vi "Start logging.vi"(3 "Custom rate":dbl=8.0, 4 "File Segmenting size (MB)":dbl=8.0, 5 "custom logging rate?":bool, 6 "FilePropertyValues":string[](array[string]), 7 "Segment Files? (F)":bool, 8 "FilePropertyNames":string[](array[string]), 9 "File Description":string, 10 "Channel paths":string[](array[string])=["Aliases/ActualRPM", "Aliases/DesiredRPM", "Aliases/EnginePower", "Aliases/EngineTemp"], 11 "Base Log File Path":path=path "C:/Users/aheim/Desktop/test.tdms") -> (0 "error out":errorcluster, 1 "Report Text":string)   [LabVIEW 2013, in "Logger.lvlib"]
uses:
  Logger.lvlib
  <vilib>/NI Veristand/Execution/DataLogging/File Conflict Operation.ctl
  <vilib>/NI Veristand/Execution/DataLogging/TDMS Channel Group.ctl
  <vilib>/NI Veristand/Execution/DataLogging/TDMS Property.ctl
  <vilib>/NI Veristand/Execution/DataLogging/TDMS Channel.ctl
  <vilib>/NI Veristand/Execution/DataLogging/Time Channel Options.ctl
  <vilib>/NI Veristand/Execution/DataLogging/New Data Logging Specification (TDMS).vi
  <vilib>/NI Veristand/Execution/DataLogging/Set Data Logging Rate (Target Rate).vi
  <vilib>/NI Veristand/Execution/DataLogging/Set Data Logging Rate (Custom Rate).vi
  <vilib>/NI Veristand/Execution/DataLogging/Set Segmenting Specification (Footprint).vi
  <vilib>/NI Veristand/Execution/DataLogging/NI_VS Data Logging API.lvlib
panel:
  in  "Gateway IP Address (\"\": localhost)":string
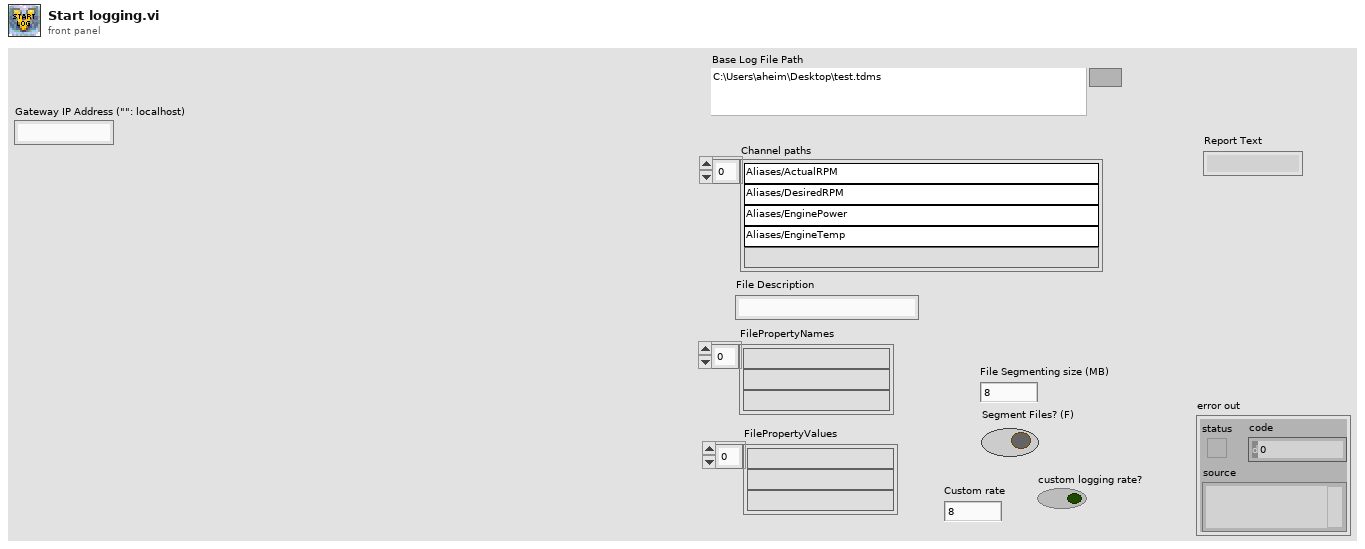
[diagram p1: front panel]
types:
  T1 = typedef "NI_VS Data Logging API.lvlib/Time Channel Options.ctl" = enum16{"No Time Channel", "Absolute Time", "System Time", "System Time - Microseconds", "Absolute Time as Double"}
  T2 = typedef "NI_VS Data Logging API.lvlib/TDMS Channel Group.ctl" = cluster{"Group Name":string, "Group Description":string, "Group Properties":T3[], "Channels":T4[], "Time Channel Options":T1, "Time Channel Name":string}
  T3 = typedef "NI_VS Data Logging API.lvlib/TDMS Property.ctl" = cluster{"Name":string, "Value":variant}
  T4 = typedef "NI_VS Data Logging API.lvlib/TDMS Channel.ctl" = cluster{"Channel Name":string, "Channel Path":string, "Channel Description":string, "Channel Properties":T3[]}
  T5 = typedef "NI_VS Data Logging API.lvlib/File Conflict Operation.ctl" = enum16{"Create Unique", "Append to Existing", "Overwrite"}
  T6 = cluster{"PropertyName":string, "PropertyValue":string}
  T7 = typedef "NI_VS Data Logging API.lvlib/IDataLogging Ref.ctl" = refnum<k24>
  T8 = typedef "NI_VS Data Logging API.lvlib/DataLoggingSpecification Ref.ctl" = refnum<k24>
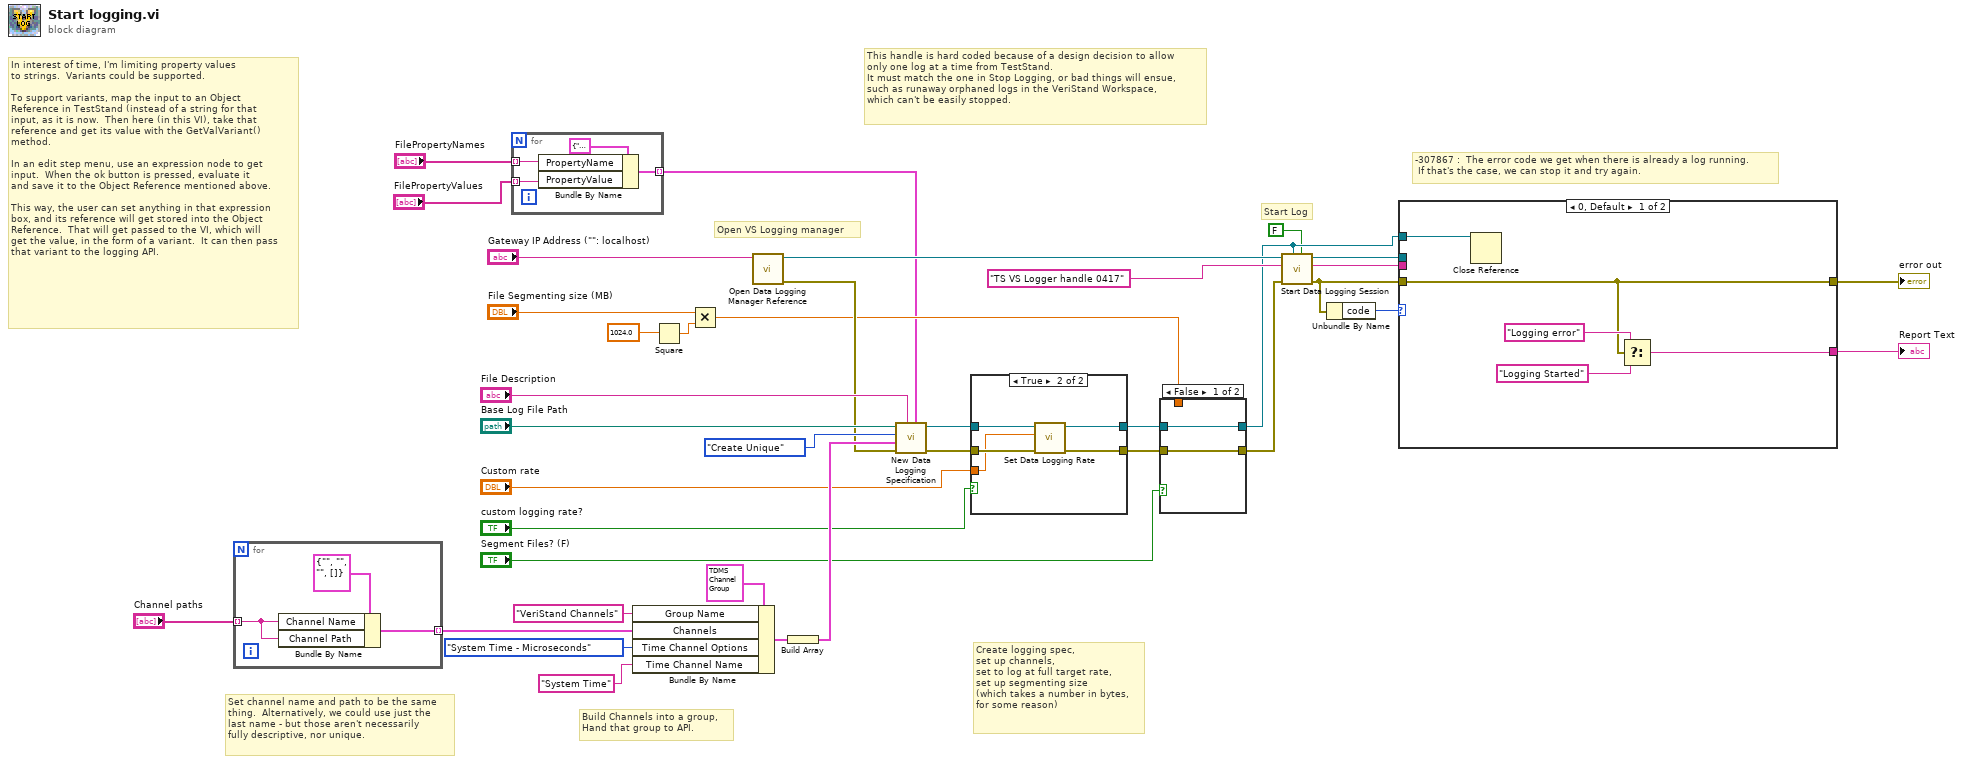
[diagram p0: block diagram]
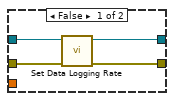
[diagram p2: hidden frame]
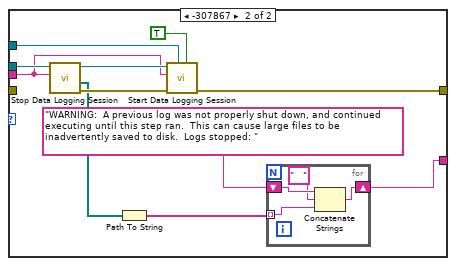
[diagram p3: hidden frame]
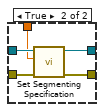
[diagram p4: hidden frame]
diagram:
  # "-307867 :  The error code we get when there is already a log running. \n If that's the case, we can stop it and try again."
  # "In interest of time, I'm limiting property values\nto strings.  Variants could be supported.\n\nTo support variants, map the input to an Object\nReference in TestStand (instead of a string for that\ninput, as it is now.  Then here (in this VI), take that\nreference and get its value with the GetValVariant()\nmethod.\n\nIn an edit step menu, use an expression node to get\ninput.  When the ok button is pressed, evaluate it\nand save it to the Object Reference mentioned above.\n\nThis way, the user can set anything in that expression\nbox, and its reference will get stored into the Object\nReference.  That will get passed to the VI, which will\nget the value, in the form of a variant.  It can then pass\nthat variant to the logging API."
  # "Set channel name and path to be the same\nthing.  Alternatively, we could use just the \nlast name - but those aren't necessarily\nfully descriptive, nor unique."
  # "Build Channels into a group,\nHand that group to API."
  # "This handle is hard coded because of a design decision to allow\nonly one log at a time from TestStand. \nIt must match the one in Stop Logging, or bad things will ensue,\nsuch as runaway orphaned logs in the VeriStand Workspace,\nwhich can't be easily stopped."
  # "Start Log"
  # "Create logging spec, \nset up channels, \nset to log at full target rate,\nset up segmenting size\n(which takes a number in bytes,\nfor some reason)"
  # "Open VS Logging manager"
  n1 = for {
    tunnel: [w40] -> w30 mode=indexing
    tunnel: "Channel paths" -> [w39] mode=indexing
    n2 = Bundle By Name(cluster=T4 {"Channel Name"="", "Channel Path"="", "Channel Description"="", "Channel Properties"=[]} ("TDMS Channel"), "Channel Name"=w39, "Channel Path"=w39) -> (w40:T4)
  }
  n3 = for {
    tunnel: "FilePropertyNames" -> [w44] mode=indexing
    tunnel: "FilePropertyValues" -> [w43] mode=indexing
    tunnel: [w42] -> w11 mode=indexing
    n4 = Bundle By Name(cluster=T6 {"PropertyName"="", "PropertyValue"=""} ("FileProperty"), "PropertyName"=w44, "PropertyValue"=w43) -> (w42:T6)
  }
  n5 = Bundle By Name(cluster=T2 {"Group Name"="", "Group Description"="", "Group Properties"=[], "Channels"=[], "Time Channel Options"=enum."No Time Channel", "Time Channel Name"="Time"} ("TDMS Channel Group"), "Group Name"="VeriStand Channels", "Channels"=w30, "Time Channel Options"=Time_Channel_Options."System Time - Microseconds", "Time Channel Name"="System Time") -> (w35:T2)
  n6 = Square(x=1024.0 ("x*y")) -> (x^2=w18:dbl)
  n7 = Multiply(x="File Segmenting size (MB)", y=w18) -> (x*y=w15:dbl)
  n8 = call <vilib>:"Open Data Logging Manager Reference.vi"("Gateway IP Address (\"\": localhost)"="Gateway IP Address (\"\": localhost)") -> ("error out"=w23:errorcluster, "Data Logging Manager Ref out"=w24:T7)  [unwired: 9 in]
  n9 = Build Array(w35) -> (w34:T2[])
  n10 = call-poly <vilib>:"New Data Logging Specification.vi"("File Properties"=w11, "File Description"="File Description", "error in (no error)"=w23, "Channel Groups"=w34, "File Conflict Operation"=File_Conflict_Operation."Create Unique", "Base Log File Path"="Base Log File Path") -> ("error out"=w27:errorcluster, "Data Logging Specification Ref out"=w26:T8)  [unwired: 4 in]
  n11 = case shown="True" "custom logging rate?" {
    tunnel: w27 -> [w49 w52]
    tunnel: w26 -> [w48 w54]
    tunnel: [w47 w53] -> w21
    tunnel: [w46 w51] -> w20
    tunnel: "Custom rate" -> [_ w50]
    frame False {
      n12 = call-poly <vilib>:"Set Data Logging Rate.vi"("error in (no error)"=w49, "Data Logging Specification Ref in"=w48) -> ("error out"=w46:errorcluster, "Data Logging Specification Ref out"=w47:T8)  [unwired: 8 in]
    }
    frame True {
      n13 = call-poly <vilib>:"Set Data Logging Rate.vi"("error in (no error)"=w52, "Custom Rate (Hz)"=w50, "Data Logging Specification Ref in"=w54) -> ("error out"=w51:errorcluster, "Data Logging Specification Ref out"=w53:T8)  [unwired: 7 in]
    }
  }
  n14 = case shown="False" "Segment Files? (F)" {
    tunnel: w21 -> [w56 w61]
    tunnel: w20 -> [w55 w60]
    tunnel: [w55 w59] -> w19
    tunnel: [w56 w58] -> w7
    tunnel: w15 -> [_ w57]
    frame False {
    }
    frame True {
      n15 = call-poly <vilib>:"Set Segmenting Specification.vi"("error in (no error)"=w60, "Size"=w57, "Data Logging Specification Ref in"=w61) -> ("error out"=w59:errorcluster, "Data Logging Specification Ref out"=w58:T8)  [unwired: 7 in]
    }
  }
  n16 = call <vilib>:"Start Data Logging Session.vi"("Close Data Logging Specification Ref (T)"=FALSE, "Data Logging Specification Ref in"=w7, "error in (no error)"=w19, "Session Name in"="TS VS Logger handle 0417" ("Logging Session Name in"), "Data Logging Manager Ref in"=w24) -> ("error out"=w6:errorcluster, "Session Name out"=w8:string, "Data Logging Manager Ref out"=w9:T7)  [unwired: 4 in]
  n17 = Unbundle By Name(w6) -> ("code"=w10:i32)
  n18 = case shown="0, Default" w10 {
    tunnel: w9 -> [_ w77]
    tunnel: w8 -> [_ w75]
    tunnel: w7 -> [w62 w68]
    tunnel: w6 -> [w64 _]
    tunnel: [w64 w73] -> w5
    tunnel: [w63 w69] -> w4
    frame 0, Default {
      n19 = Close Reference(reference=w62) -> ()  [unwired: 1 in, 1 out]
      n20 = Select(t="Logging error" ("Report Text"), s=w64, f="Logging Started" ("Report Text")) -> (s? t:f=w63:string)
    }
    frame -307867 {
      n21 = call <vilib>:"Stop Data Logging Session.vi"("Session Name in"=w75, "Data Logging Manager Ref in"=w77) -> ("error out"=w74:errorcluster, "Log File Paths"=w70:path[], "Data Logging Manager Ref out"=w76:T7)  [unwired: 7 in]
      n22 = Path To String(path=w70) -> (string=w71:string[])
      n23 = call <vilib>:"Start Data Logging Session.vi"("Close Data Logging Specification Ref (T)"=TRUE, "Data Logging Specification Ref in"=w68, "error in (no error)"=w74, "Session Name in"=w75, "Data Logging Manager Ref in"=w76) -> ("error out"=w73:errorcluster)  [unwired: 4 in, 2 out]
      n24 = for {
        shift-right: [w78] -> w69
        shift-left: "WARNING:  A previous log was not properly shut down, and continued executing until this step ran.  This can cause large files to be inadvertently saved to disk.  Logs stopped: " -> [w81]
        tunnel: w71 -> [w80] mode=indexing
        n25 = Concatenate Strings(w81, "   " ("string"), w80) -> (w78:string)
      }
    }
  }
  "error out" <- w5
  "Report Text" <- w4
